vi "zk.vi"(0 "p12":dbl, 5 "p21":dbl, 7 "uk":dbl) -> (8 "zk":dbl)   [LabVIEW 2017]
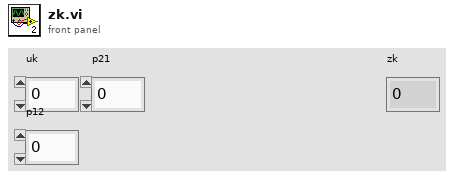
[diagram p1: front panel]
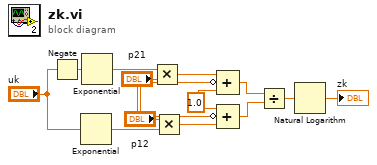
[diagram p0: block diagram]
diagram:
  w7 = 1.0 ("value")
  n1 = Negate(x="uk") -> (-x=w13:dbl)
  n2 = Exponential(1:"uk") -> (0:w10:dbl)
  n3 = Exponential(1:w13) -> (0:w11:dbl)
  n4 = Multiply(x=w11, y="p21") -> (x*y=w9:dbl)
  n5 = Multiply(x="p12", y=w10) -> (x*y=w5:dbl)
  n6 = Compound Arithmetic op=ADD(w9, invert "p12", w7) -> (w4:dbl)
  n7 = Compound Arithmetic op=ADD(w7, invert "p21", w5) -> (w3:dbl)
  n8 = Divide(x=w4, y=w3) -> (x/y=w2:dbl)
  n9 = Natural Logarithm(1:w2) -> (0:→"zk":dbl)
